vi "IO_18v7Driver.vi"(10 "Inputs":T3, 11 "Reply In":string) -> (0 "Tx Buf Out":string, 2 "Outputs":T2)   [LabVIEW 2024]
uses:
  Control Definitions/DEF_18v7DriverInputs.ctl
  Control Definitions/Def_Status18v7.ctl
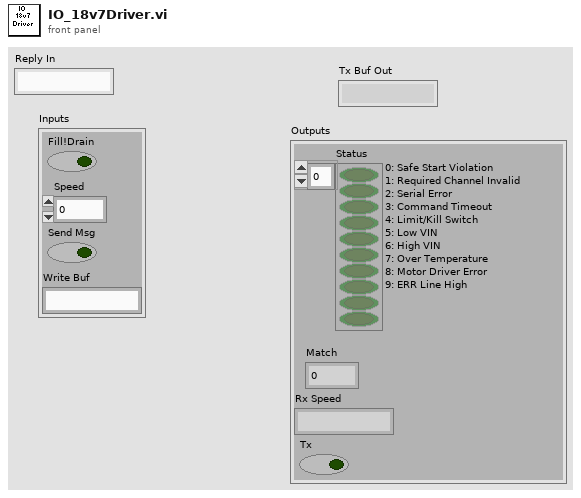
[diagram p1: front panel]
types:
  T1 = typedef "Def_Status18v7.ctl" = bool[]
  T2 = cluster{"Status":T1, "Match":i32, "Rx Speed":string, "Tx":bool}
  T3 = typedef "DEF_18v7DriverInputs.ctl" = cluster{"Fill!Drain":bool, "Speed":i16, "Send Msg":bool, "Write Buf":string}
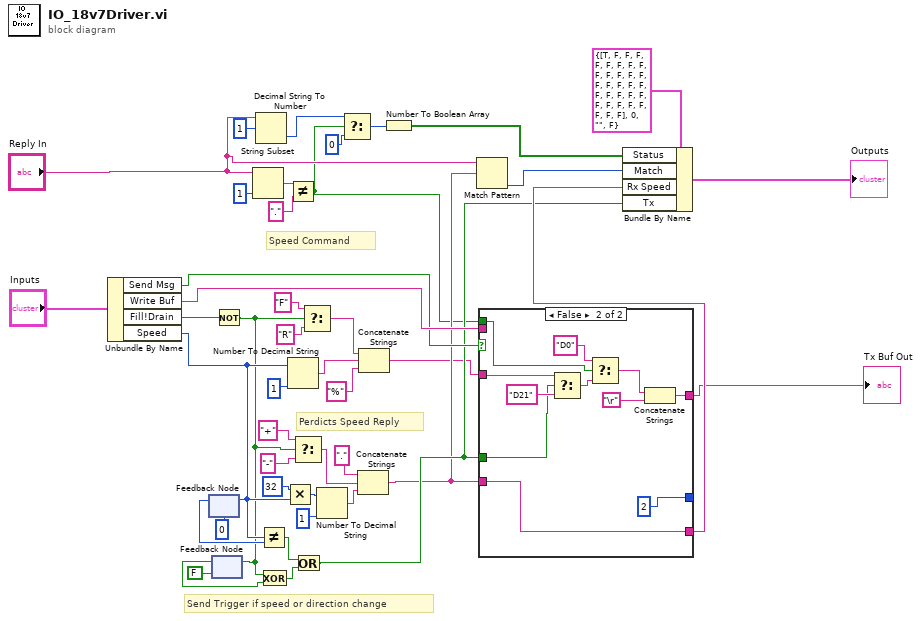
[diagram p0: block diagram]
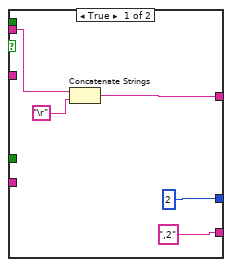
[diagram p2: hidden frame]
diagram:
  # "Send Trigger if speed or direction change"
  # "Speed Command"
  # "Perdicts Speed Reply"
  n1 = Unbundle By Name("Inputs") -> ("Send Msg"=w41:bool, "Write Buf"=w42:string, "Fill!Drain"=w2:bool, "Speed"=w43:i16)
  n2 = feedback #1(i16 0 ("Speed")) -> (w14:i16)
  n3 = feedback-in #1(w43) -> ()
  n4 = feedback #2(FALSE ("Fill!Drain")) -> (w22:bool)
  n5 = Not(x=w2) -> (.not. x?=w1:bool)
  n6 = feedback-in #2(w1) -> ()
  n7 = String Subset(string="Reply In", length (rest)=1 ("length (rest)")) -> (substring=w27:string)  [unwired: 1 in]
  n8 = Decimal String To Number(string="Reply In", offset=1) -> (number=w30:i32)  [unwired: 1 in, 1 out]
  n9 = Not Equal?(x=w43, y=w14) -> (x != y?=w23:bool)
  n10 = Exclusive Or(1:w22, 2:w1) -> (0:w24:bool)
  n11 = Multiply(x=32, y=w43) -> (x*y=w9:i32)
  n12 = Not Equal?(x=w27, y=".") -> (x != y?=w32:bool)
  n13 = Number To Decimal String(number=w43, width (-)=i16 1) -> (decimal integer string=w19:string)
  n14 = Select(t="+", s=w1, f="-") -> (s? t:f=w11:string)
  n15 = Or(x=w23, y=w24) -> (x .or. y?=w38:bool)
  n16 = Select(t="F", s=w1, f="R") -> (s? t:f=w18:string)
  n17 = Number To Decimal String(number=w9, width (-)=i16 1) -> (decimal integer string=w10:string)
  n18 = Select(t=w30, s=w32, f=0) -> (s? t:f=w29:i32)
  n19 = Concatenate Strings(".", w11, w10) -> (w33:string)
  n20 = Concatenate Strings(w18, w19, "%" ("string")) -> (w3:string)
  n21 = Number To Boolean Array(number=w29) -> (Boolean array=w35:bool[])
  n22 = Match Pattern(string="Reply In", regular expression=w33) -> (offset past match=w37:i32)  [unwired: 1 in, 3 out]
  n23 = case shown="False" w41 {
    tunnel: w32 -> [_ w50]
    tunnel: w3 -> [_ w55]
    tunnel: [w48 w59] -> w4
    tunnel: [2 2] -> _
    tunnel: w33 -> [_ w57]
    tunnel: [",2" w57] -> w44
    tunnel: w38 -> [_ w53]
    tunnel: w42 -> [w45 _]
    frame True {
      n24 = Concatenate Strings(w45, "\r") -> (w48:string)
    }
    frame False {
      n25 = Select(t=w55, s=w53, f="D21" ("write buffer 2")) -> (s? t:f=w52:string)
      n26 = Select(t="D0" ("write buffer 2"), s=w50, f=w52) -> (s? t:f=w56:string)
      n27 = Concatenate Strings(w56, "\r") -> (w59:string)
    }
  }
  "Tx Buf Out" <- w4
  n28 = Bundle By Name(cluster=T2 {"Status"=[TRUE, FALSE, FALSE, FALSE, FALSE, FALSE, FALSE, FALSE, FALSE, FALSE, FALSE, FALSE, FALSE, FALSE, FALSE, FALSE, FALSE, FALSE, FALSE, FALSE, FALSE, FALSE, FALSE, FALSE, FALSE, FALSE, FALSE, FALSE, FALSE, FALSE, FALSE, FALSE], "Match"=0, "Rx Speed"="", "Tx"=FALSE} ("Cluster"), "Status"=w35, "Match"=w37, "Rx Speed"=w44, "Tx"=w38) -> (→"Outputs":T2)
